vi "shutDownCamera.vi"(8 "error in (no error)":errorcluster, 10 "Log in":refnum<class "Log.lvclass">, 11 "CameraController in":refnum<class "CameraController.lvclass">) -> (0 "error out":errorcluster, 2 "Log out":refnum<class "Log.lvclass">, 3 "CameraController out":refnum<class "CameraController.lvclass">)   [LabVIEW 2009, in "Hardware.lvlib" / "Channels.lvlib" / "CameraController.lvclass"]
uses:
  CameraController.lvclass
  Tools/Log.lvclass
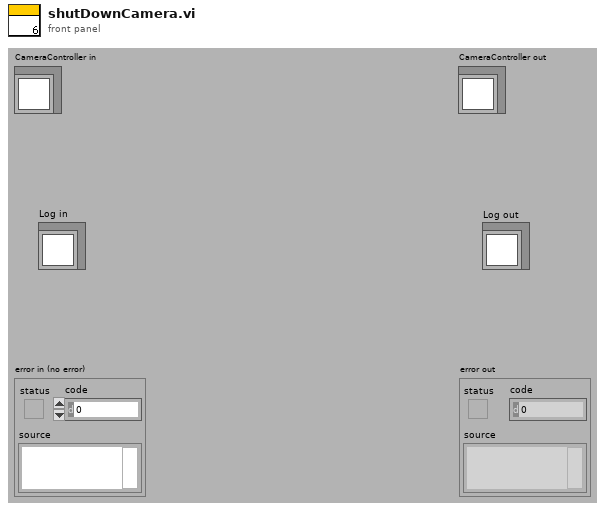
[diagram p1: front panel]
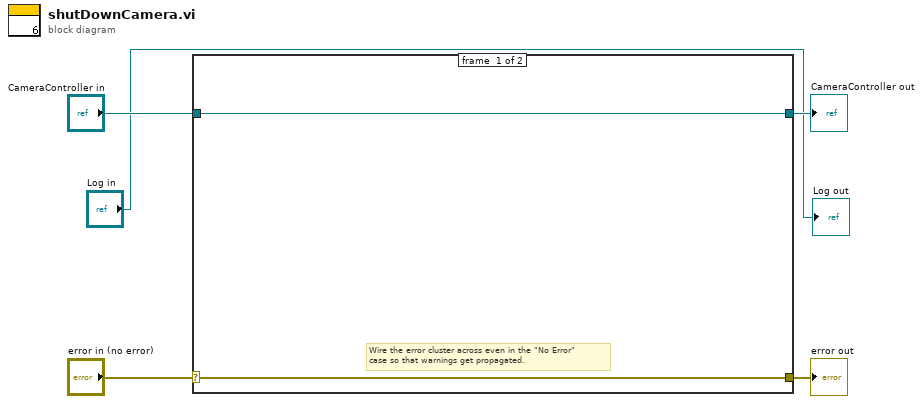
[diagram p0: block diagram]
diagram:
  n1 = case shown="No Error" "error in (no error)" {
    selector: "error in (no error)" -> [w7 w9]
    tunnel: [w7 w9] -> w4
    tunnel: [w6 w8] -> w2
    tunnel: "CameraController in" -> [w6 w8]
    frame #0 {
      # "Wire the error cluster across even in the \"No Error\"\ncase so that warnings get propagated."
    }
    frame #1 {
    }
  }
  "error out" <- w4
  "CameraController out" <- w2
  "Log out" <- "Log in"
